vi "Generate Event.vi"(0 "Include NMR Data":bool) -> ()   [LabVIEW 2019]
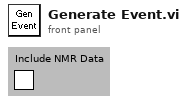
[diagram p1: front panel]
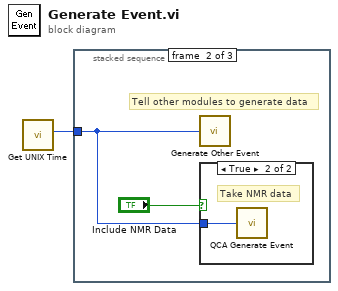
[diagram p0: block diagram]
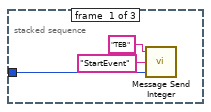
[diagram p2: hidden frame]
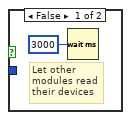
[diagram p3: hidden frame]
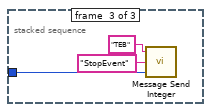
[diagram p4: hidden frame]
diagram:
  n1 = call "Get UNIX Time.vi"() -> ("UNIX seconds"=w1:i32)  [unwired: 10 in, 1 out]
  n2 = stacked-sequence {
    tunnel: w1 -> [w2 w5 w9]
    frame #0 {
      n3 = call "Message Send Integer.vi"("Value"=w2, "Parameter"="StartEvent", "Destination"="TEB") -> ()
    }
    frame #1 {
      # "Tell other modules to generate data"
      n4 = call "Generate Other Event.vi"("Event Number"=w5) -> ()
      n5 = case shown="True" "Include NMR Data" {
        tunnel: w5 -> [_ w8]
        frame False {
          # "Let other modules read their devices"
          n6 = Wait (ms)(milliseconds to wait=u32 3000) -> ()  [unwired: 1 out]
        }
        frame True {
          # "Take NMR data"
          n7 = call "QCA Generate Event.vi"("Event Number"=w8) -> ()
        }
      }
    }
    frame #2 {
      n8 = call "Message Send Integer.vi"("Value"=w9, "Parameter"="StopEvent", "Destination"="TEB") -> ()
    }
  }
